vi "Read Num.vi"(8 "error in (no error)":errorcluster, 10 "Ctl Refnum":refnum<vi>, 11 "Worksheet Reference":refnum<k7>) -> (0 "error out":errorcluster)   [LabVIEW 2015]
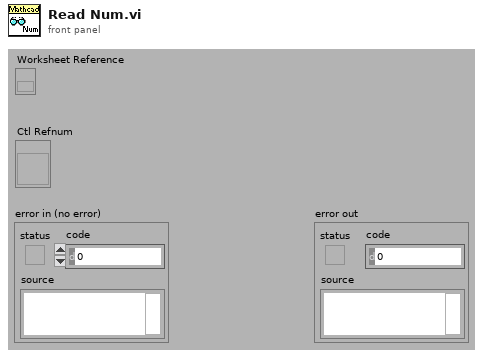
[diagram p1: front panel]
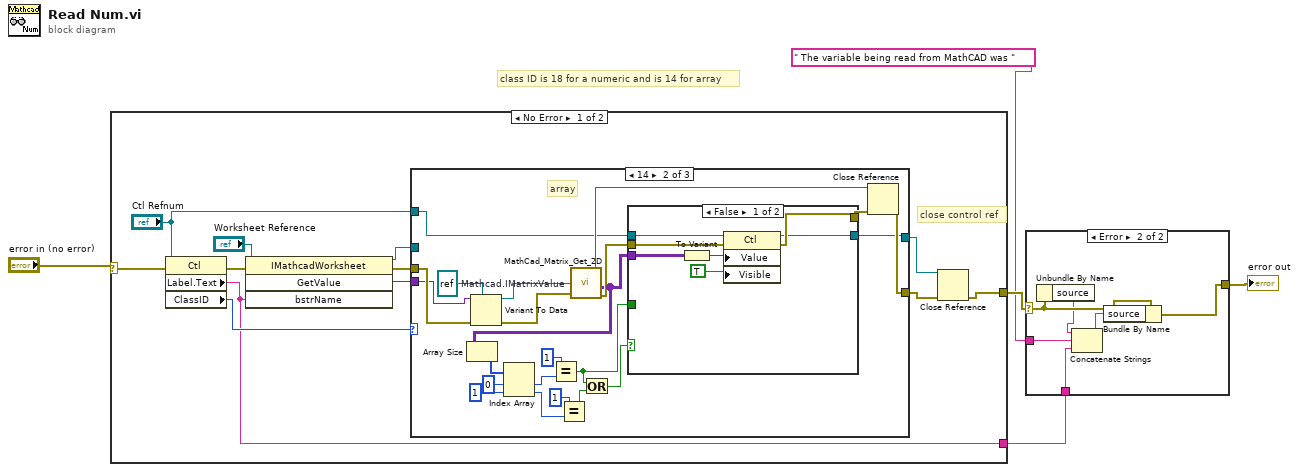
[diagram p0: block diagram]
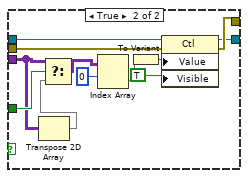
[diagram p4: hidden frame]
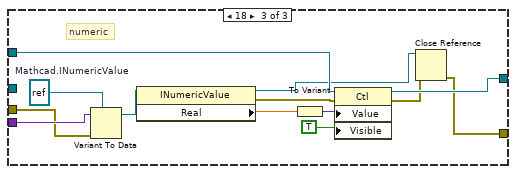
[diagram p5: hidden frame]
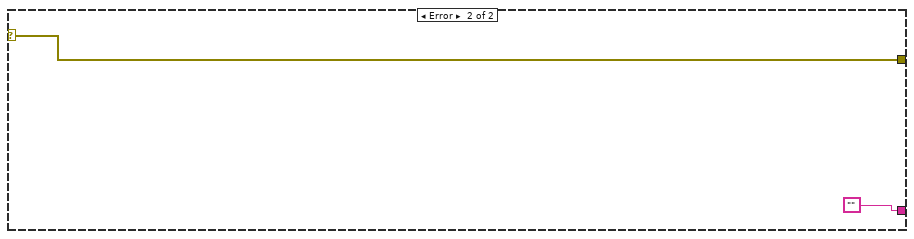
[diagram p6: hidden frame]
diagram:
  # "class ID is 18 for a numeric and is 14 for array"
  n1 = case shown="No Error" "error in (no error)" {
    selector: "error in (no error)" -> [w16 w75]
    tunnel: [w8 w75] -> w4
    tunnel: [w6 ""] -> w2
    frame No Error {
      # "close control ref"
      n2 = property class="Ctl"(reference="Ctl Refnum", error in=w16) -> (error out=w15:errorcluster, "Label.Text"=w6:string, "ClassID"=w14:u32)  [unwired: 1 out]
      n3 = invoke class="IMathcadWorksheet" method="GetValue"(reference="Worksheet Reference", error in=w15, "bstrName"=w6) -> (reference out=w11:refnum<k7>, error out=w12:errorcluster, "GetValue"=w13:variant)  [unwired: 1 in, 1 out]
      n4 = case shown="14" w14 {
        tunnel: [w19 w32 w70] -> w7
        tunnel: w13 -> [_ w40 w69]
        tunnel: w12 -> [w18 w41 w68]
        tunnel: w11 -> [_ _ _]
        tunnel: "Ctl Refnum" -> [w19 w20 w65]
        tunnel: [w18 w37 w62] -> w9
        frame 0, Default {
        }
        frame 14 {
          w39 = refnum<k7> refnum  # Mathcad.IMatrixValue
          # "array"
          n5 = Variant To Data(error in=w41, type=w39, Variant=w40) -> (data=w38:refnum<k7>, error out=w33:errorcluster)
          n6 = call "MathCad_Matrix_Get_2D.vi"("Mathcad.IMatrixValue Refnum"=w38, "error out 2"=w33) -> ("Mathcad.IMatrixValue Refnum"=w36:refnum<k7>, "Array"=w31:variant[][], "error out"=w35:errorcluster)  [unwired: 2 in]
          n7 = Array Size(array=w31) -> (size(s)=w30:i32[])
          n8 = Index Array(array=w30, index #1=0 ("index"), index #2=1 ("index")) -> (element #1=w27:i32, element #2=w24:i32)
          n9 = Equal?(x=1 ("index"), y=w27) -> (x = y?=w21:bool)
          n10 = Equal?(x=1 ("index"), y=w24) -> (x = y?=w23:bool)
          n11 = Or(x=w21, y=w23) -> (x .or. y?=w22:bool)
          n12 = case shown="False" w22 {
            tunnel: w35 -> [w47 w59]
            tunnel: [w46 w58] -> w34
            tunnel: [w45 w57] -> w32
            tunnel: w20 -> [w44 w56]
            tunnel: w31 -> [w43 w51]
            tunnel: w21 -> [_ w53]
            frame False {
              n13 = To Variant(anything=w43) -> (Variant=w48:variant)
              n14 = property class="Ctl"(reference=w44, error in=w47, "Value"=w48, "Visible"=TRUE) -> (reference out=w45:refnum<vi>, error out=w46:errorcluster)
            }
            frame True {
              n15 = Transpose 2D Array(2D array=w51) -> (transposed array=w50:variant[][])
              n16 = Select(t=w51, s=w53, f=w50) -> (s? t:f=w52:variant[][])
              n17 = Index Array(array=w52, index (row)=0) -> (element=w55:variant[])  [unwired: 1 in]
              n18 = To Variant(anything=w55) -> (Variant=w60:variant)
              n19 = property class="Ctl"(reference=w56, error in=w59, "Value"=w60, "Visible"=TRUE) -> (reference out=w57:refnum<vi>, error out=w58:errorcluster)
            }
          }
          n20 = Close Reference(reference=w36, error in (no error)=w34) -> (error out=w37:errorcluster)
        }
        frame 18 {
          w67 = refnum<k7> refnum  # Mathcad.INumericValue
          # "numeric"
          n21 = Variant To Data(error in=w68, type=w67, Variant=w69) -> (data=w66:refnum<k7>)  [unwired: 1 out]
          n22 = property class="INumericValue"(reference=w66) -> (reference out=w64:refnum<k7>, error out=w71:errorcluster, "Real"=w73:dbl)  [unwired: 1 in]
          n23 = To Variant(anything=w73) -> (Variant=w72:variant)
          n24 = property class="Ctl"(reference=w65, error in=w71, "Value"=w72, "Visible"=TRUE) -> (reference out=w70:refnum<vi>, error out=w63:errorcluster)
          n25 = Close Reference(reference=w64, error in (no error)=w63) -> (error out=w62:errorcluster)
        }
      }
      n26 = Close Reference(reference=w7, error in (no error)=w9) -> (error out=w8:errorcluster)
    }
    frame Error {
    }
  }
  n27 = case shown="Error" w4 {
    selector: w4 -> [w76 w82]
    tunnel: [w76 w77] -> w3
    tunnel: w2 -> [_ w79]
    tunnel: " The variable being read from MathCAD was " ("string") -> [_ w78]
    frame No Error {
    }
    frame Error {
      n28 = Unbundle By Name(w82) -> ("source"=w81:string)
      n29 = Concatenate Strings(w81, w78, w79) -> (w80:string)
      n30 = Bundle By Name(cluster=w82, "source"=w80) -> (w77:errorcluster)
    }
  }
  "error out" <- w3
